vi "Send Message.vi"(0 "VISA Session In":refnum<visa-resource-name>="OXYMAT", 1 "Target Address":u8=16 format="%.0x", 2 "Source Address":u8=208 format="%.0x", 7 "Command":string, 11 "error in (no error)":errorcluster) -> (4 "VISA Session Out":refnum<visa-resource-name>, 8 "ACK?":bool, 15 "error out":errorcluster)   [LabVIEW 2020, in "Siemens ELAN.lvlib"]
doc: "Lower-level VI which assembles and sends a message, encoded using the Siemens ELAN protocol, to the COM port specified by the VISA session. Returns a boolean indicating that the addressed device provided the ACK response.\n\n$Revision:: 0 $\n$Modtime:: yy-mm-dd hh:mm $\n$Author:: Dboyd $"
uses:
  Siemens ELAN.lvlib
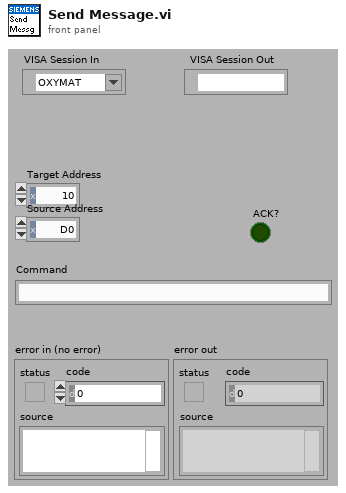
[diagram p1: front panel]
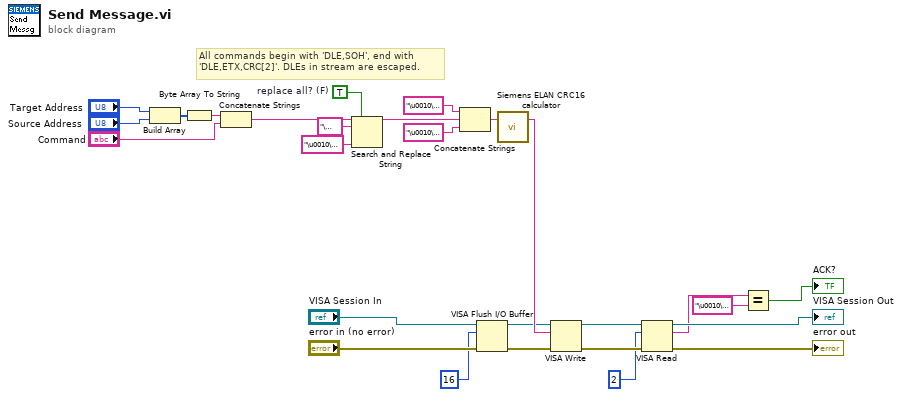
[diagram p0: block diagram]
diagram:
  w3 = TRUE  # replace all? (F)
  # "All commands begin with 'DLE,SOH', end with\n'DLE,ETX,CRC[2]'. DLEs in stream are escaped."
  n1 = Build Array("Target Address", "Source Address") -> (w23:u8[])
  n2 = Byte Array To String(unsigned byte array=w23) -> (string=w15:string)
  n3 = Concatenate Strings(w15, "Command") -> (w5:string)
  n4 = Search and Replace String(replace all?=w3, input string=w5, search string="\u0010", replace string="\u0010\u0010" ("replace string (\"\")")) -> (result string=w4:string)  [unwired: 4 in, 3 out]
  n5 = Concatenate Strings("\u0010\u0001" ("DLE,SOH"), w4, "\u0010\u0003" ("DLE,ETX")) -> (w16:string)
  n6 = VISA Flush I/O Buffer(VISA resource name="VISA Session In", mask (16)=u16 16, error in (no error)="error in (no error)") -> (VISA resource name out=w12:refnum<visa-resource-name>, error out=w10:errorcluster)
  n7 = call "Siemens ELAN CRC16 calculator.vi"("Input String"=w16) -> ("String with CRC16"=w18:string)  [unwired: 1 in, 1 out]
  n8 = VISA Write(VISA resource name=w12, write buffer=w18, error in (no error)=w10) -> (VISA resource name out=w25:refnum<visa-resource-name>, error out=w24:errorcluster)  [unwired: 1 out]
  n9 = VISA Read(VISA resource name=w25, byte count=u32 2, error in (no error)=w24) -> (VISA resource name out=→"VISA Session Out":refnum<visa-resource-name>, read buffer=w7:string, error out=→"error out":errorcluster)  [unwired: 1 out]
  n10 = Equal?(x=w7, y="\u0010\u0006") -> (x = y?=→"ACK?":bool)
